vi "ex_WriteToOpenTDMFile.vi"(4 "error if check fails":bool, 5 "File path in":path, 6 "check time attributes":bool, 7 "write ddt attr":bool, 8 "error in (no error)":errorcluster, 9 "Signals":waveform(dbl)[](array[waveform]), 10 "file params":T2 {"Flags"."time preference" items=["Absolute", "Relative"]; "Flags"."x_columns" items=["None", "One", "Multiple"]; "origin time" format="%<%X\n%x>T"}, 11 "append info in":T1) -> (0 "error out":errorcluster, 1 "open file was used":bool, 2 "bytes written":i32, 3 "append info out":T1)   [LabVIEW 2020]
uses:
  storage/Storage.llb/__savePropTime.vi
  storage/Storage.llb/_commitObject.vi
  storage/Storage.llb/Set Property (String).vi
  express/express input/ExFileReadBlock.llb/ex_ReadFileParams.ctl
  express/express output/ExFileWriteBlock.llb/ex_WriteFileParams.ctl
  ex_appendInfoTDM.ctl
panel:
  out "storage refnums (channel) out":refnum<k20>[](array[refnum])
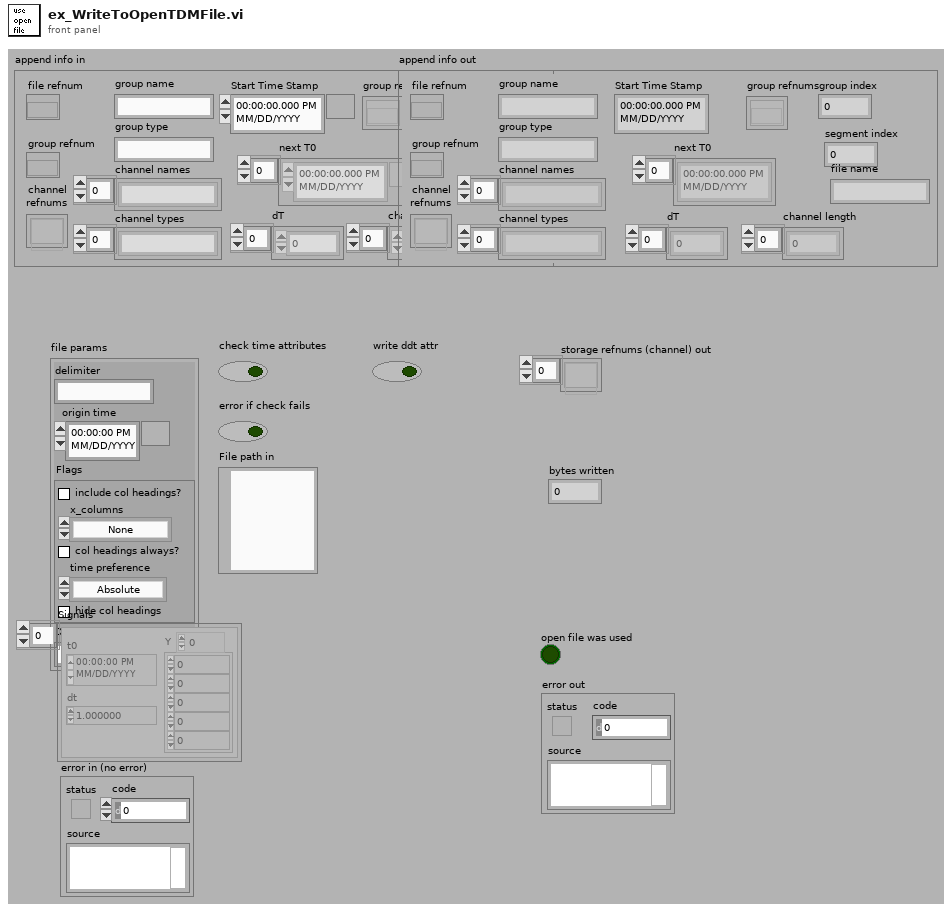
[diagram p1: front panel]
types:
  T1 = typedef "ex_appendInfoTDM.ctl" = cluster{"channel\nrefnums":refnum<k20>[], "channel names":string[], "channel types":string[], "file refnum":refnum<k20>, "group refnum":refnum<k20>, "group name":string, "group type":string, "next T0":timestamp[], "dT":dbl[], "Start Time Stamp":timestamp, "channel length":u32[], "group index":u32, "group refnums":refnum<k20>[], "file name":string, "segment index":u32}
  T2 = typedef "ex_WriteFileParams.ctl" = cluster{"delimiter":string, "origin time":timestamp, "Flags":T3, "Decimal Separator":string}
  T3 = typedef "ex_ReadFileParams.ctl" = cluster{"include col headings?":bool, "x_columns":u16, "col headings always?":bool, "time preference":u16, "hide col headings":bool}
  T4 = cluster{"Start Timestamp":timestamp, "Timestamp":timestamp, "Relative Time?":bool, "X Dimension":string, "Signal Name":string, "Y Units":string, "X0":timestamp, "dX":dbl, "nPoints":i32}[]
  T5 = typedef "ex_WaveformAttribsPlus.ctl" = cluster{"Start Timestamp":timestamp, "Timestamp":timestamp, "Relative Time?":bool, "X Dimension":string, "Signal Name":string, "Y Units":string, "X0":timestamp, "dX":dbl, "nPoints":i32}
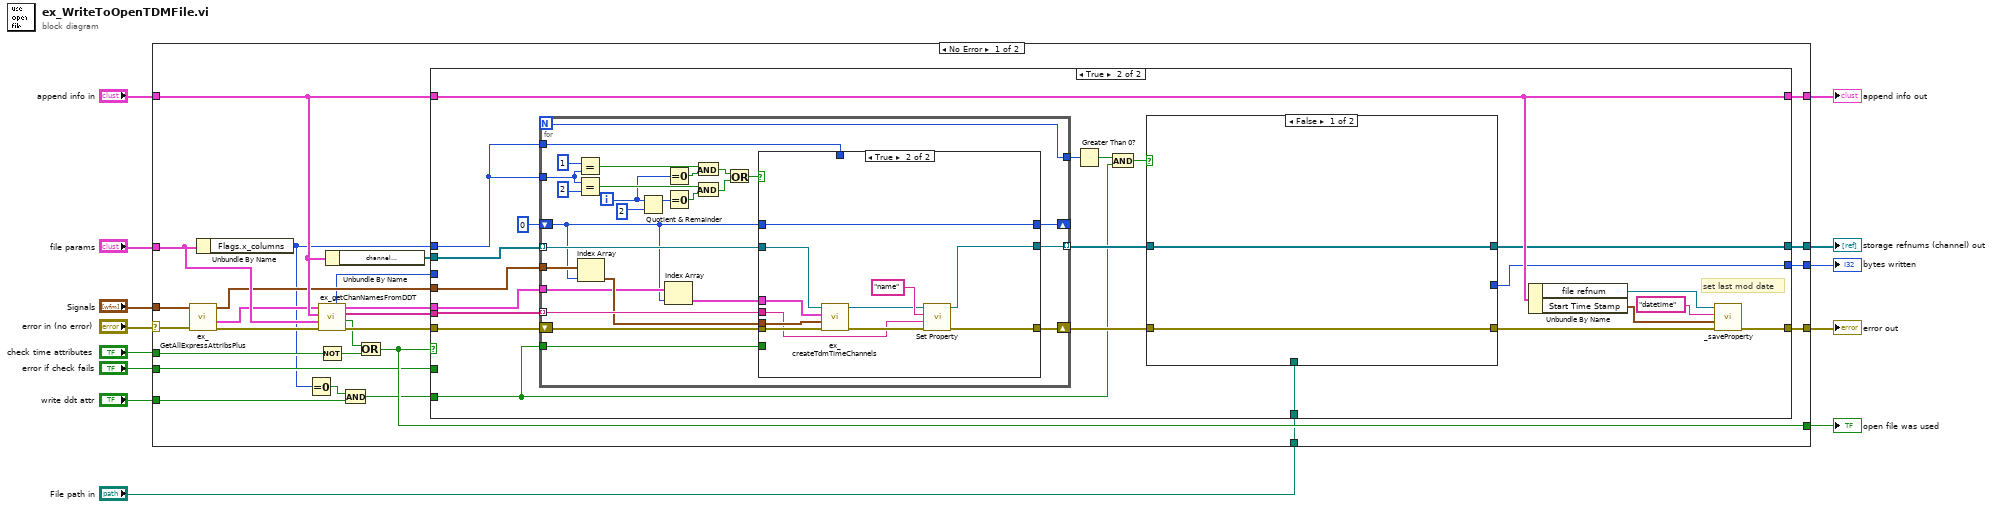
[diagram p0: block diagram]
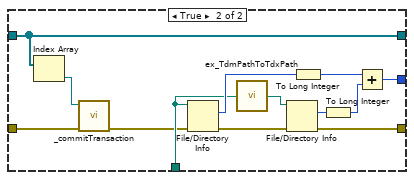
[diagram p3: hidden frame]
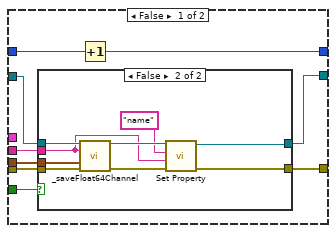
[diagram p4: hidden frame]
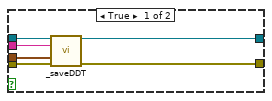
[diagram p5: hidden frame]
diagram:
  n1 = case shown="No Error" "error in (no error)" {
    selector: "error in (no error)" -> [w28 w141]
    tunnel: [w39 w141] -> w13
    tunnel: [w38 _] -> w12
    tunnel: [w37 _] -> w11
    tunnel: "Signals" -> [w36 _]
    tunnel: "append info in" -> [w32 w142]
    tunnel: [w31 w142] -> w8
    tunnel: "file params" -> [w30 _]
    tunnel: [w27 _] -> w6
    tunnel: "check time attributes" -> [w25 _]
    tunnel: "error if check fails" -> [w24 _]
    tunnel: "write ddt attr" -> [w16 _]
    tunnel: "File path in" -> [w14 _]
    frame No Error {
      n2 = call "ex_GetAllExpressAttribsPlus.vi"("error in"=w28, "Signals in"=w36) -> ("error out"=w20:errorcluster, "All Express Wave Attributes Plus"=w22:T4, "Signals out"=w21:waveform(dbl)[])  [unwired: 7 out]
      n3 = Unbundle By Name(w30) -> ("Flags.x_columns"=w18:u16)
      n4 = Equal To 0?(x=w18) -> (x = 0?=w17:bool)
      n5 = call "ex_getChanNamesFromDDT.vi"("error in (no error)"=w20, "file params"=w30, "append info in"=w32, "Express Wave Attributes in"=w22) -> ("error out"=w33:errorcluster, "channels match"=w29:bool, "channel names"=w34:string[], "Express Wave Attributes out"=w35:T5[], "error code"=w19:i32)  [unwired: 2 in, 1 out]
      n6 = Not(x=w25) -> (.not. x?=w26:bool)
      n7 = Unbundle By Name(w32) -> ("channel\nrefnums"=w23:refnum<k20>[])
      n8 = And(x=w17, y=w16) -> (x .and. y?=w15:bool)
      n9 = Or(x=w29, y=w26) -> (x .or. y?=w27:bool)
      n10 = case shown="True" w27 {
        tunnel: w23 -> [_ w57]
        tunnel: w33 -> [w40 w53]
        tunnel: [w40 w63] -> w39
        tunnel: [_ w50] -> w38
        tunnel: [_ w52] -> w37
        tunnel: w34 -> [_ w54]
        tunnel: w18 -> [_ w58]
        tunnel: w21 -> [_ w56]
        tunnel: w35 -> [_ w55]
        tunnel: w32 -> [w41 w62]
        tunnel: [w41 w62] -> w31
        tunnel: w24 -> [_ _]
        tunnel: w19 -> [_ _]
        tunnel: w15 -> [_ w43]
        tunnel: w14 -> [_ w42]
        frame False {
        }
        frame True {
          # "set last mod date"
          n11 = for {
            N -> [w82]
            tunnel: [w82] -> w47
            shift-right: [w103] -> w46
            shift-left: w53 -> [w105]
            tunnel: w57 -> [w104] mode=indexing
            tunnel: [w101] -> w48 mode=indexing
            tunnel: w55 -> [w97]
            tunnel: w54 -> [w102] mode=indexing
            tunnel: w58 -> [w89]
            shift-right: [w100] -> _
            shift-left: 0 -> [w96]
            tunnel: w56 -> [w99]
            tunnel: w58 -> [w81]
            tunnel: w43 -> [w80]
            i -> [w88]
            n12 = Equal?(x=1, y=w89) -> (x = y?=w86:bool)
            n13 = Equal?(x=w89, y=2) -> (x = y?=w91:bool)
            n14 = Index Array(array=w99, index=w96) -> (element=w98:waveform(dbl))
            n15 = Quotient & Remainder(x=w88, y=2) -> (x-y*floor(x/y)=w94:i32)  [unwired: 1 out]
            n16 = Index Array(array=w97, index=w96) -> (element=w79:T5)
            n17 = Equal To 0?(x=w88) -> (x = 0?=w87:bool)
            n18 = Equal To 0?(x=w94) -> (x = 0?=w92:bool)
            n19 = And(x=w86, y=w87) -> (x .and. y?=w84:bool)
            n20 = And(x=w91, y=w92) -> (x .and. y?=w85:bool)
            n21 = Or(x=w84, y=w85) -> (x .or. y?=w83:bool)
            n22 = case shown="True" w83 {
              tunnel: w79 -> [_ w140]
              tunnel: w105 -> [w114 w139]
              tunnel: [w113 w133] -> w103
              tunnel: w104 -> [w112 w138]
              tunnel: [w111 w131] -> w101
              tunnel: w102 -> [w110 w130]
              tunnel: w96 -> [w108 w137]
              tunnel: [w109 w137] -> w100
              tunnel: w98 -> [w107 w136]
              tunnel: w81 -> [_ _]
              tunnel: w80 -> [w106 _]
              frame False {
                n23 = case shown="False" w106 {
                  tunnel: w114 -> [w120 w128]
                  tunnel: [w119 w124] -> w113
                  tunnel: w112 -> [w118 w129]
                  tunnel: [w117 w123] -> w111
                  tunnel: w110 -> [w116 w121]
                  tunnel: w107 -> [w115 w127]
                  frame True {
                    n24 = call "_saveDDT.vi"("Data object in"=w118, "Name"=w116, "Values"=w115, "error in (no error)"=w120) -> ("Data object out"=w117:refnum<k20>, "error out"=w119:errorcluster)  [unwired: 5 in, 5 out]
                  }
                  frame False {
                    n25 = call "_saveFloat64Channel.vi"("Data object in"=w129, "Name"=w121, "Values"=w127, "error in (no error)"=w128) -> ("Data object out"=w126:refnum<k20>, "error out"=w125:errorcluster)  [unwired: 5 in, 5 out]
                    n26 = call-poly "Set Property.vi"("error in (no error)"=w125, "Value"=w121, "Property name"="name", "storage refnum"=w126) -> ("error out"=w124:errorcluster, "storage refnum out"=w123:refnum<k20>)  [unwired: 2 in, 4 out]
                  }
                }
                n27 = Increment(x=w108) -> (x+1=w109:i32)
              }
              frame True {
                n28 = call "ex_createTdmTimeChannels.vi"("error in (no error)"=w139, "waveform"=w136, "All Express Wave Attributes Plus"=w140, "Data object in"=w138) -> ("error out"=w134:errorcluster, "Data object out"=w132:refnum<k20>)  [unwired: 2 out]
                n29 = call-poly "Set Property.vi"("error in (no error)"=w134, "Value"=w130, "Property name"="name", "storage refnum"=w132) -> ("error out"=w133:errorcluster, "storage refnum out"=w131:refnum<k20>)  [unwired: 2 in, 4 out]
              }
            }
          }
          n30 = Greater Than 0?(x=w47) -> (x > 0?=w45:bool)
          n31 = And(x=w45, y=w43) -> (x .and. y?=w44:bool)
          n32 = case shown="False" w44 {
            tunnel: [w65 w78] -> w51
            tunnel: w46 -> [w65 w69]
            tunnel: [_ w77] -> w52
            tunnel: w48 -> [w64 w67]
            tunnel: [w64 w67] -> w50
            tunnel: w42 -> [_ w70]
            frame False {
            }
            frame True {
              n33 = Index Array(array=w67) -> (element=w66:refnum<k20>)  [unwired: 1 in]
              n34 = call-poly "_commitTransaction.vi"("error in (no error)"=w69, "storage refnum"=w66) -> ("error out"=w68:errorcluster)  [unwired: 5 out]
              n35 = File/Directory Info(path=w70, error in=w68) -> (size=w71:i64, error out=w76:errorcluster)  [unwired: 5 out]
              n36 = call "ex_TdmPathToTdxPath.vi"("TDM path"=w70) -> ("TDX path"=w75:path)
              n37 = File/Directory Info(path=w75, error in=w76) -> (size=w72:i64, error out=w78:errorcluster)  [unwired: 5 out]
              n38 = To Long Integer(number=w71) -> (32bit integer=w73:i32)
              n39 = To Long Integer(number=w72) -> (32bit integer=w74:i32)
              n40 = Add(x=w73, y=w74) -> (x+y=w77:i32)
            }
          }
          n41 = Unbundle By Name(w62) -> ("file refnum"=w61:refnum<k20>, "Start Time Stamp"=w59:timestamp)
          n42 = call-poly "_saveProperty.vi"("error in (no error)"=w51, "Value"=w59, "Property name"="datetime", "storage refnum"=w61) -> ("error out"=w63:errorcluster)  [unwired: 1 in, 6 out]
        }
      }
    }
    frame Error {
    }
  }
  "error out" <- w13
  "storage refnums (channel) out" <- w12
  "open file was used" <- w6
  "bytes written" <- w11
  "append info out" <- w8
